vi "get_image_path_for splitting.vi"(11 "Image/ File Directory":path) -> (3 "Array":path[](array[path]))   [LabVIEW 2024]
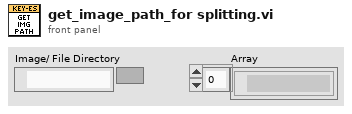
[diagram p1: front panel]
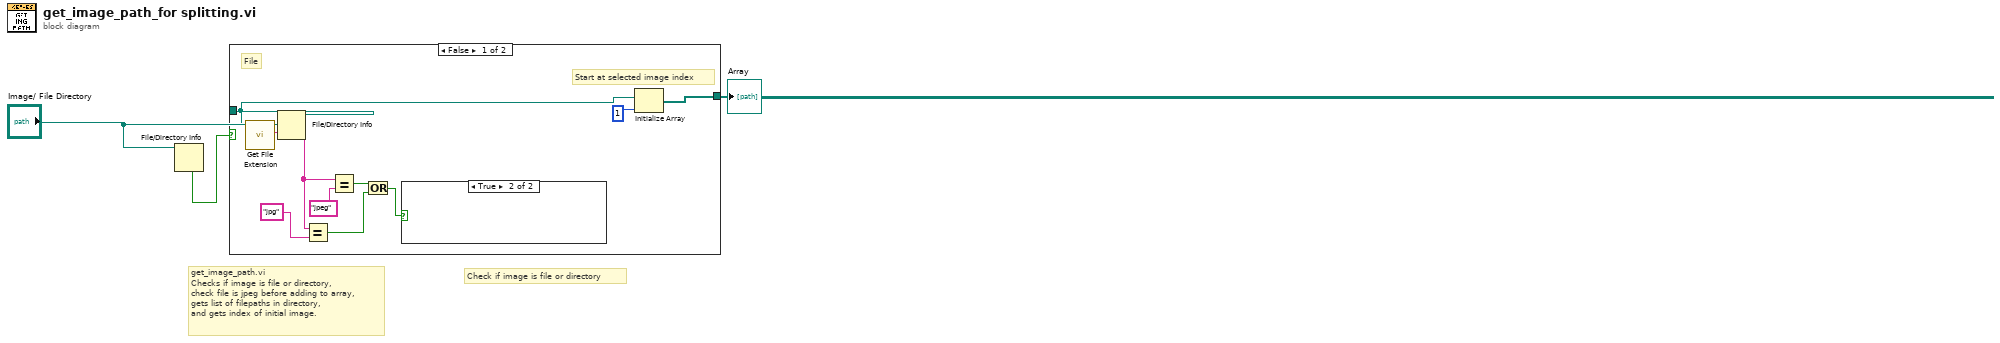
[diagram p0: block diagram]
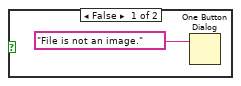
[diagram p2: hidden frame]
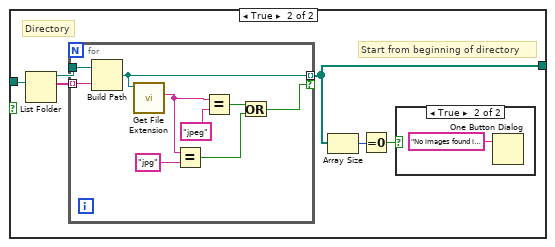
[diagram p3: hidden frame]
diagram:
  # "get_image_path.vi\nChecks if image is file or directory,\ncheck file is jpeg before adding to array,\ngets list of filepaths in directory,\nand gets index of initial image."
  # "Check if image is file or directory"
  n1 = File/Directory Info(path="Image/ File Directory") -> (directory=w4:bool)  [unwired: 1 in, 6 out]
  n2 = File/Directory Info(path="Image/ File Directory") -> (path out=w2:path)  [unwired: 1 in, 6 out]
  n3 = case shown="False" w4 {
    tunnel: w2 -> [w5 w20]
    tunnel: [w6 w17] -> w1
    frame False {
      # "File"
      # "Start at selected image index"
      n4 = call <vilib>:"Get File Extension.vi"("file"=w5) -> ("lowercase file extension"=w8:string)  [unwired: 6 in, 4 out]
      n5 = Equal?(x=w8, y="jpg") -> (x = y?=w11:bool)
      n6 = Equal?(x=w8, y="jpeg") -> (x = y?=w12:bool)
      n7 = Or(x=w12, y=w11) -> (x .or. y?=w9:bool)
      n8 = case shown="True" w9 {
        frame False {
          n9 = One Button Dialog(message="File is not an image.") -> ()  [unwired: 1 in, 1 out]
        }
        frame True {
        }
      }
      n10 = Initialize Array(w5, 1 ("dimension size")) -> (w6:path[])
    }
    frame True {
      # "Directory"
      # "Start from beginning of directory"
      n11 = List Folder(path=w20) -> (path out=w18:path, filenames=w19:string[])  [unwired: 3 in, 2 out]
      n12 = for {
        tunnel: w19 -> [w30] mode=indexing
        tunnel: w18 -> [w29]
        tunnel: [w27] -> w17 mode=indexing if=w22
        n13 = Build Path(base path=w29, name or relative path=w30) -> (appended path=w27:path)
        n14 = call <vilib>:"Get File Extension.vi"("file"=w27) -> ("lowercase file extension"=w25:string)  [unwired: 6 in, 4 out]
        n15 = Equal?(x=w25, y="jpg") -> (x = y?=w23:bool)
        n16 = Equal?(x=w25, y="jpeg") -> (x = y?=w24:bool)
        n17 = Or(x=w24, y=w23) -> (x .or. y?=w22:bool)
      }
      n18 = Array Size(array=w17) -> (size(s)=w16:i32)
      n19 = Equal To 0?(x=w16) -> (x = 0?=w15:bool)
      n20 = case shown="True" w15 {
        frame False {
        }
        frame True {
          n21 = One Button Dialog(message="No images found in directory.") -> ()  [unwired: 1 in, 1 out]
        }
      }
    }
  }
  "Array" <- w1
